vi "p4.5.vi"() -> ()   [LabVIEW 2020]
uses:
  <vilib>/Analysis/2dsp.llb/Decimate (continuous, DBL).vi
  <vilib>/Analysis/NI_AALPro.lvlib
panel:
  out "Tono original":dbl[](graph)
  out "Tono diezmado M=2":dbl[](graph)
  in  "fs AD (Hz)":dbl=50000.0 min=0.0 max=50000.0
  in  "fs DA (Hz)":dbl=-1.0 min=-1.0 max=50000.0
  in  "Canal AD":tag="myDAQ1/audioInputLeft"
  in  "Canal DA":tag="myDAQ1/audioOutputLeft"
  out "error out":errorcluster
  in  "Número muestras":i32
  in  "stop":bool
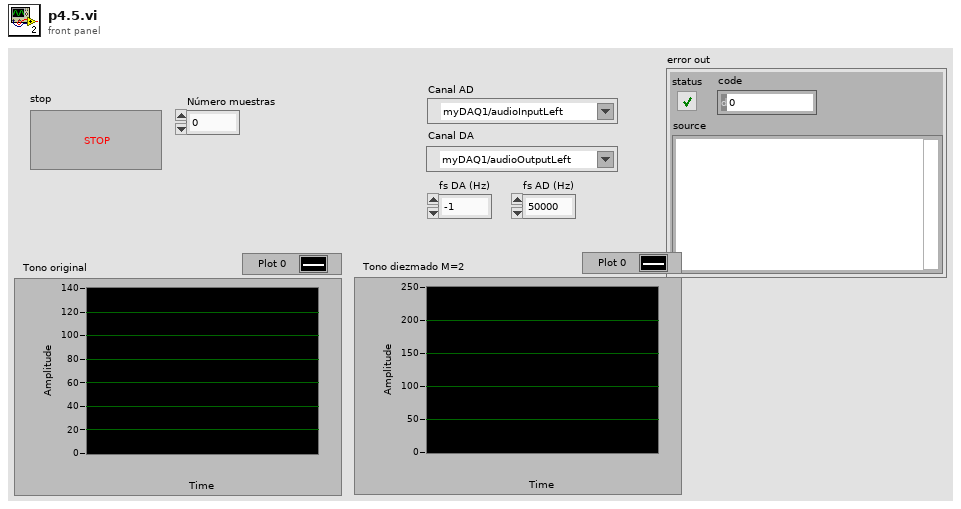
[diagram p1: front panel]
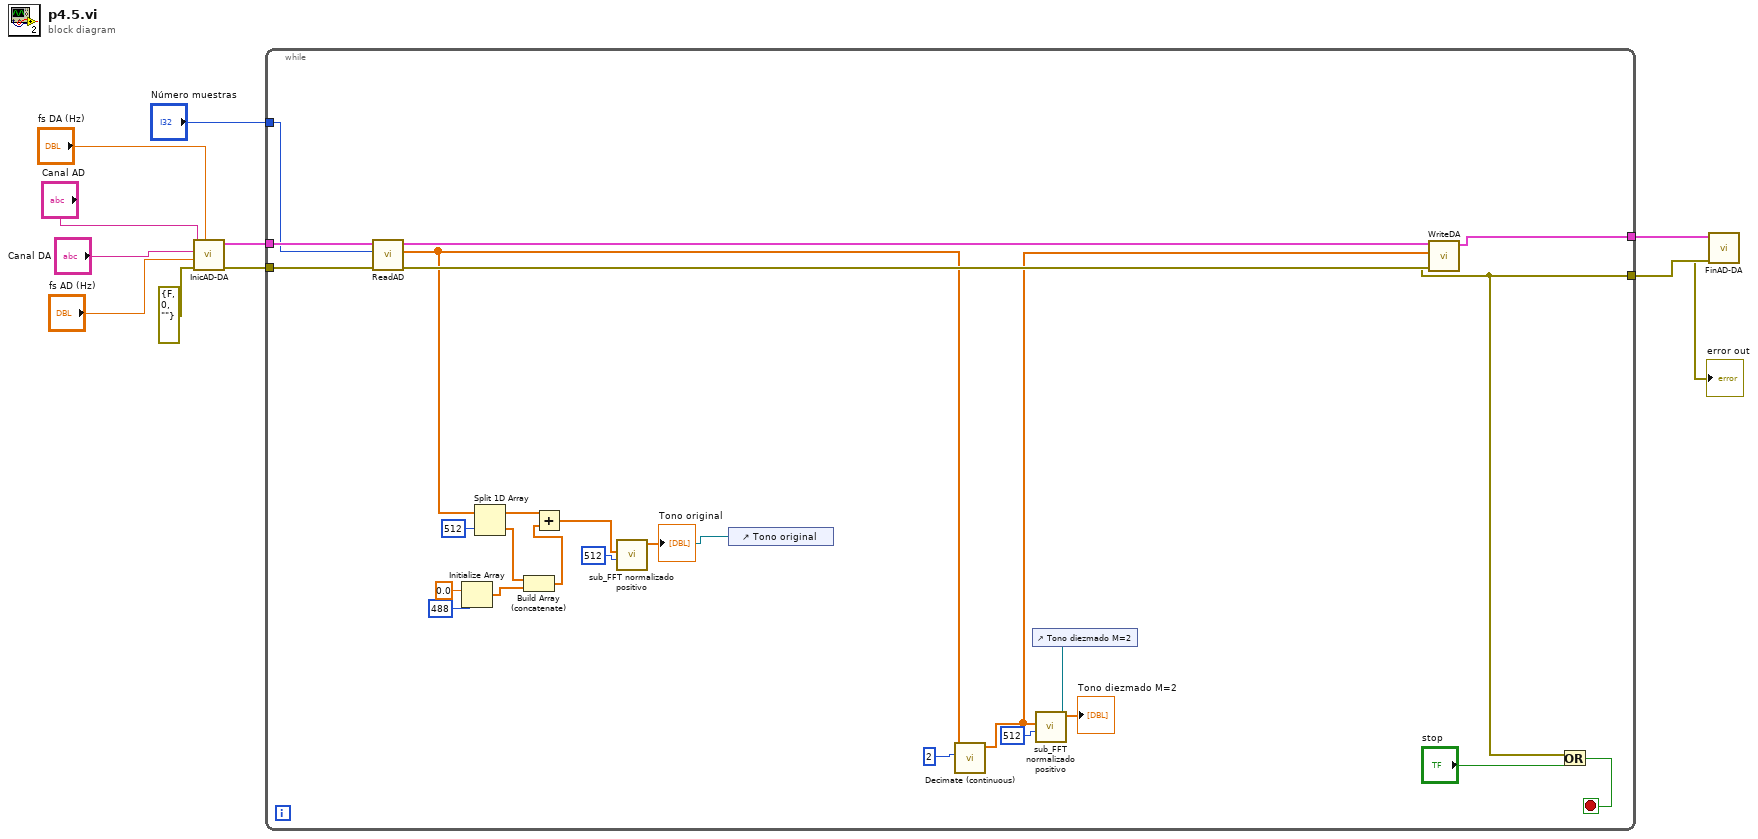
[diagram p0: block diagram]
diagram:
  n1 = call <userlib>:"InicAD-DA.vi"("fs DA (Hz)"="fs DA (Hz)", "error in"=errorcluster {"status"=FALSE, "code"=0, "source"=""}, "fs AD (Hz)"="fs AD (Hz)", "Canal DA"="Canal DA", "Canal AD"="Canal AD") -> ("error out"=w9:errorcluster, "Tarea Out"=w10:cluster{"AD":refnum<k21>, "DA":refnum<k21>})  [unwired: 5 in]
  n2 = while {
    tunnel: w10 -> [w36]
    tunnel: w9 -> [w35]
    tunnel: [w14] -> w8
    tunnel: "Número muestras" -> [w31]
    tunnel: [w13] -> w1
    stop <- w33 stop-if-true
    n3 = call <userlib>:"ReadAD.vi"("error in"=w35, "numero de muestras"=w31, "Tarea In"=w36) -> ("error out"=w34:errorcluster, "Datos"=w23:dbl[], "Tarea Out"=w37:cluster{"AD":refnum<k21>, "DA":refnum<k21>})  [unwired: 6 in]
    n4 = Initialize Array(0.0 ("element"), 488 ("dimension size")) -> (w20:dbl[])
    n5 = Split 1D Array(array=w23, index=512) -> (first subarray=w21:dbl[], second subarray=w17:dbl[])
    n6 = Build Array (concatenate)(w17, w20) -> (w16:dbl[])
    n7 = Add(x=w21, y=w16) -> (x+y=w15:dbl[])
    n8 = control-ref of="Tono original"() -> (w24:refnum<vi>)
    n9 = call "sub_FFT normalizado positivo.vi"("FFT size"=512, "Array in"=w15, "WaveformGraph in"=w24) -> ("Array out"=→"Tono original":dbl[])  [unwired: 8 in]
    n10 = call-poly <vilib>:"Decimate (continuous).vi"("decimating factor"=2, "X"=w23) -> ("Decimated Array"=w12:dbl[])  [unwired: 8 in, 1 out]
    n11 = control-ref of="Tono diezmado M=2"() -> (w29:refnum<vi>)
    n12 = call "sub_FFT normalizado positivo.vi"("FFT size"=512, "Array in"=w12, "WaveformGraph in"=w29) -> ("Array out"=→"Tono diezmado M=2":dbl[])  [unwired: 8 in]
    n13 = call <userlib>:"WriteDA.vi"("error in"=w34, "Datos"=w12, "Tarea In"=w37) -> ("error out"=w14:errorcluster, "Tarea Out"=w13:cluster{"AD":refnum<k21>, "DA":refnum<k21>})  [unwired: 7 in]
    n14 = Or(x=w14, y="stop") -> (x .or. y?=w33:bool)
  }
  n15 = call <userlib>:"FinAD-DA.vi"("error in"=w8, "Tarea In"=w1) -> ("error out"=→"error out":errorcluster)  [unwired: 9 in]
